vi "Read from File.vi"(8 "error in (no error)":errorcluster, 10 "INI Ref":T1, 11 "Mouse Macro in":refnum<class "Mouse Macro.lvclass">) -> (0 "error out":errorcluster, 2 "INI Ref out":T1, 3 "Mouse Macro out":refnum<class "Mouse Macro.lvclass">)   [LabVIEW 2020, in "MacroAssert.lvlib" / "Mouse Macro.lvclass"]
uses:
  Mouse Macro.lvclass
  C:/Users/acasalen/Documents/LabVIEW Data/Projects/MacroAssert/source/Classes/Step/Step.lvclass
  Macro Step/Macro Step.lvclass
  <vilib>/Utility/config.llb/NI_LVConfig.lvlib
  <vilib>/Utility/config.llb/Read Key (I32).vi
  MacroAssert.lvlib
  <vilib>/Utility/config.llb/Read Key (Boolean).vi
  <vilib>/Utility/config.llb/Config Data RefNum.ctl
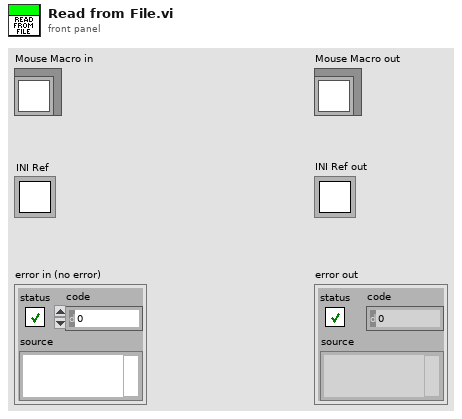
[diagram p1: front panel]
types:
  T1 = typedef "NI_LVConfig.lvlib/Config Data RefNum.ctl" = refnum<k1>
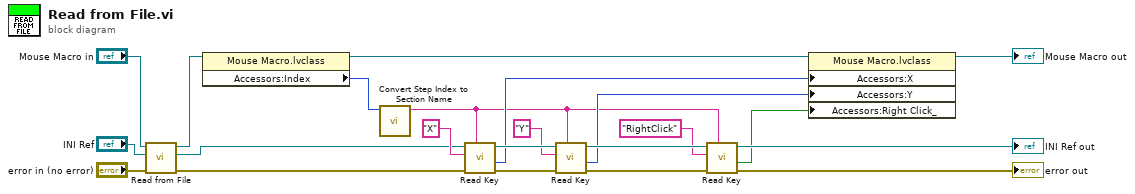
[diagram p0: block diagram]
diagram:
  n1 = call-parent "Read from File.vi"("error in (no error)"="error in (no error)", "INI Ref"="INI Ref", "Macro Step in"="Mouse Macro in") -> ("error out"=w11:errorcluster, "INI Ref out"=w10:T1, "Macro Step out"=w18:refnum<class "Mouse Macro.lvclass">)  [unwired: 6 in]
  n2 = property class="Mouse Macro.lvclass"(reference=w18) -> (reference out=w3:refnum<class "Mouse Macro.lvclass">, "Accessors:Index"=w2:i32)  [unwired: 1 in, 1 out]
  n3 = call "Convert Step Index to Section Name.vi"("Step Index"=w2) -> ("Section Name"=w1:string)  [unwired: 10 in]
  n4 = call-poly <vilib>:"Read Key.vi"("section"=w1, "error in (no error)"=w11, "key"="X", "refnum"=w10) -> ("error out"=w16:errorcluster, "value"=w12:i32, "refnum out"=w15:T1)  [unwired: 4 in, 1 out]
  n5 = call-poly <vilib>:"Read Key.vi"("section"=w1, "error in (no error)"=w16, "key"="Y", "refnum"=w15) -> ("error out"=w8:errorcluster, "value"=w5:i32, "refnum out"=w22:T1)  [unwired: 4 in, 1 out]
  n6 = call-poly <vilib>:"Read Key.vi"("section"=w1, "error in (no error)"=w8, "key"="RightClick", "refnum"=w22) -> ("error out"=→"error out":errorcluster, "value"=w4:bool, "refnum out"=→"INI Ref out":T1)  [unwired: 4 in, 1 out]
  n7 = property class="Mouse Macro.lvclass"(reference=w3, "Accessors:X"=w12, "Accessors:Y"=w5, "Accessors:Right Click_"=w4) -> (reference out=→"Mouse Macro out":refnum<class "Mouse Macro.lvclass">)  [unwired: 1 in, 1 out]
